vi "VCS Get Velocity Regulator Gain.vi"(8 "error in (no error)":errorcluster, 11 "axis in":cluster{"keyHandle":u32, "nodeId":u16}={"keyHandle"=0, "nodeId"=1}) -> (0 "error out":errorcluster, 2 "gains":cluster{"p-Gain":u16, "i-Gain":u16}, 3 "axis out":cluster{"keyHandle":u32, "nodeId":u16}={"keyHandle"=0, "nodeId"=1})   [LabVIEW 2010]
doc: "<B>VCS Get Velocity Regulator Gain</B> reads all velocity regulator gains."
uses:
  Resources/EposCmd.dll
  Resources/EposCmd64.dll
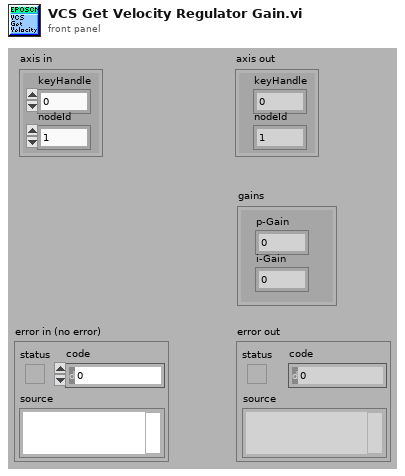
[diagram p1: front panel]
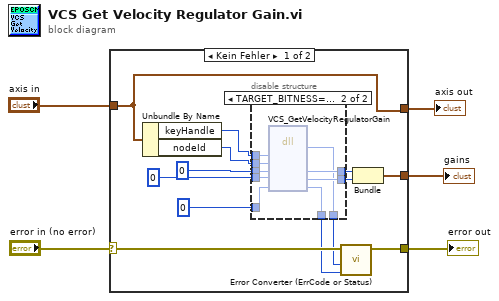
[diagram p0: block diagram]
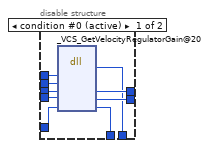
[diagram p2: hidden frame]
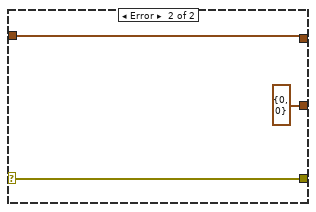
[diagram p3: hidden frame]
diagram:
  n1 = case shown="Kein Fehler" "error in (no error)" {
    selector: "error in (no error)" -> [w18 w39]
    tunnel: [w17 w39] -> w4
    tunnel: "axis in" -> [w13 w38]
    tunnel: [w13 w38] -> w2
    tunnel: [w10 cluster{"pP":u16, "pI":u16} {"pP"=0, "pI"=0}] -> w1
    frame No Error {
      n2 = Unbundle By Name(w13) -> ("keyHandle"=w15:u32, "nodeId"=w14:u16)
      n3 = disable-structure shown="TARGET_BITNESS==64" {
        disable-tunnel: [w27 w36] -> w16
        disable-tunnel: w15 -> [w26 w35]
        disable-tunnel: w14 -> [w25 w34]
        disable-tunnel: [w24 w33] -> w12
        disable-tunnel: [w23 w32] -> w11
        disable-tunnel: u16 0 ("pP") -> [w22 w31]
        disable-tunnel: u16 0 ("pI") -> [w21 w30]
        disable-tunnel: u32 0 ("pErrorCode") -> [w20 w29]
        disable-tunnel: [w19 w28] -> w6
        frame condition #0 (active) {
          n4 = dll-call lib="C:/Sources/LabView/maxon EPOS/Resources/EposCmd.*" fn="_VCS_GetVelocityRegulatorGain@20"("KeyHandle"=w26, "NodeId"=w25, "pP"=w22, "pI"=w21, "pErrorCode"=w20) -> (w19:i32, "pP"=w24:u16, "pI"=w23:u16, "pErrorCode"=w27:u32)  [unwired: 5 in, 2 out]
        }
        frame condition #1 {
          n5 = dll-call lib="C:/setup/Resources/EposCmd64.*" fn="VCS_GetVelocityRegulatorGain" ("EposCmd.dll:_VCS_GetVelocityRegulatorGain@20")("KeyHandle"=w35, "NodeId"=w34, "pP"=w31, "pI"=w30, "pErrorCode"=w29) -> ("Rückgabetyp"=w28:i32, "pP"=w33:u16, "pI"=w32:u16, "pErrorCode"=w36:u32)  [unwired: 5 in, 2 out]
        }
      }
      n6 = call "Error Converter (ErrCode or Status).vi"("error code"=w16, "return type"=w6, "error in (no error)"=w18) -> ("error out"=w17:errorcluster)  [unwired: 7 in]
      n7 = Bundle("pP"=w12, "pI"=w11) -> (w10:cluster{"pP":u16, "pI":u16})  [unwired: 1 in]
    }
    frame Error {
    }
  }
  "error out" <- w4
  "gains" <- w1
  "axis out" <- w2
